vi "PanelClose.vi"(8 "error in (no error)":errorcluster, 11 "PLC_Module in":refnum<class "PLC_Module.lvclass">) -> (0 "error out":errorcluster, 3 "PLC_Module out":refnum<class "PLC_Module.lvclass">)   [LabVIEW 2025, in "PLC_Module.lvlib" / "PLC_Module.lvclass"]
uses:
  PLC_Module.lvclass
  PLC_Module.lvclass/PLC_Module.ctl
  Msg.ctl
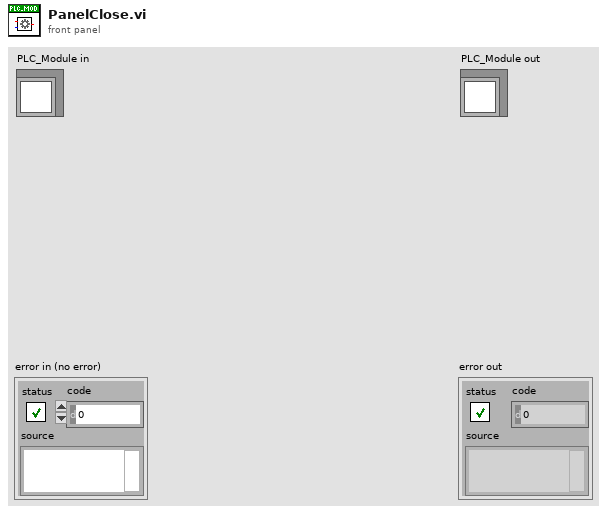
[diagram p1: front panel]
types:
  T1 = typedef "Msg.ctl" = string
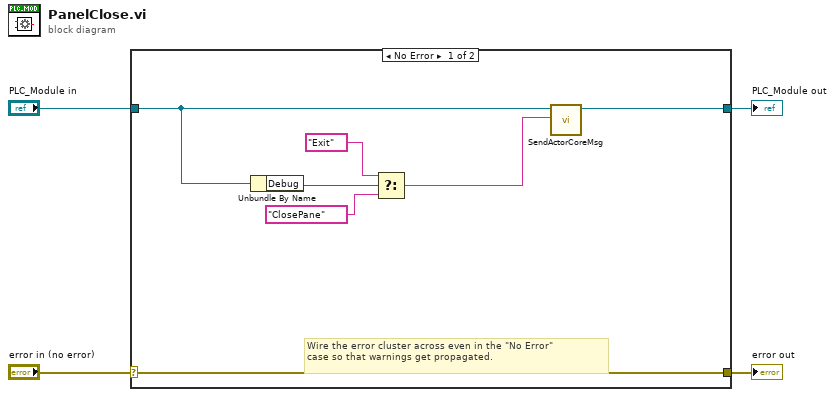
[diagram p0: block diagram]
diagram:
  n1 = case shown="No Error" "error in (no error)" {
    selector: "error in (no error)" -> [w11 w13]
    tunnel: [w11 w13] -> w3
    tunnel: [w10 w12] -> w1
    tunnel: "PLC_Module in" -> [w9 w12]
    frame No Error {
      # "Wire the error cluster across even in the \"No Error\"\ncase so that warnings get propagated."
      n2 = Unbundle By Name(w9) -> ("Debug"=w8:bool)
      n3 = Select(t=T1 "Exit" ("Msg"), s=w8, f=T1 "ClosePane" ("Msg")) -> (s? t:f=w5:T1)
      n4 = call "SendActorCoreMsg.vi"("Msg"=w5, "PLC_Module in"=w9) -> ("PLC_Module out"=w10:refnum<class "PLC_Module.lvclass">)  [unwired: 8 in, 1 out]
    }
    frame Error {
    }
  }
  "error out" <- w3
  "PLC_Module out" <- w1
